vi "Dequeue Data.vi"(8 "error in (no error)":errorcluster, 11 "queue in":refnum<queue>) -> (0 "error out":errorcluster, 1 "Data":variant, 2 "Message":string, 3 "queue out":refnum<queue>)   [LabVIEW 2014, in "Queues Lib.lvlib"]
uses:
  Queues Lib.lvlib
  Queues Message Type Def.ctl
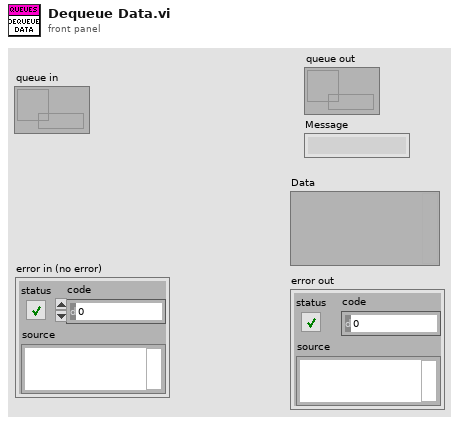
[diagram p1: front panel]
types:
  T1 = typedef "Queues Lib.lvlib/Queues Message Type Def.ctl" = cluster{"Message":string, "Data":variant}
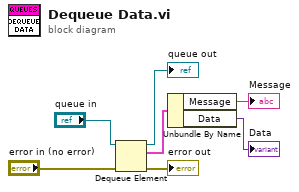
[diagram p0: block diagram]
diagram:
  n1 = Dequeue Element(queue="queue in", error in (no error)="error in (no error)") -> (queue out=→"queue out":refnum<queue>, element=w7:T1, error out=→"error out":errorcluster)  [unwired: 1 in, 1 out]
  n2 = Unbundle By Name(w7) -> ("Message"=→"Message":string, "Data"=→"Data":variant)
